vi "PS Control Test (FPGA).vi"() -> ()   [LabVIEW 2019]
uses:
  <vilib>/eio/EIONode/EIONode.xnode
  <vilib>/rvi/eio/common/nirviEmuTemplateMethod_errors.vi
panel:
  in  "RMC/DIO63":bool
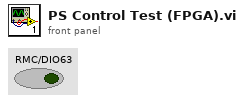
[diagram p1: front panel]
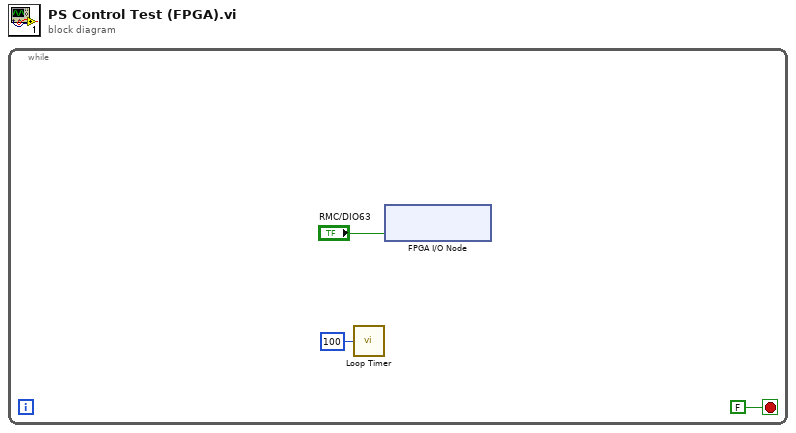
[diagram p0: block diagram]
diagram:
  n1 = while {
    stop <- FALSE stop-if-true
    n2 = call "Loop Timer"("Count(uSec)"=u32 100) -> ()  [unwired: 1 out]
    n3 = xnode "FPGA I/O Node"("RMC/DIO63"="RMC/DIO63") -> ()  [unwired: 1 in, 1 out]
  }
